vi "add_customize_control.vi"(8 "error in":errorcluster, 9 "Control Path":path, 10 "Control Position on BD":cluster{"Left":i32, "Top":i32}, 11 "VI Ref In":refnum<vi>) -> (0 "error out":errorcluster, 2 "Ctl Refnum":refnum<vi>, 3 "VI Ref Out":refnum<vi>)   [LabVIEW 2018]
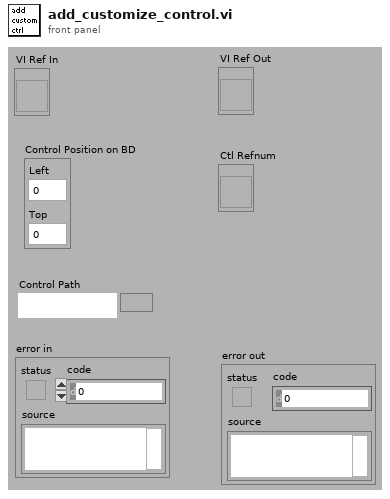
[diagram p1: front panel]
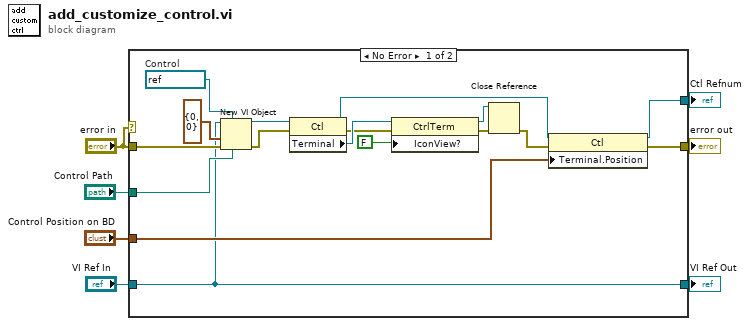
[diagram p0: block diagram]
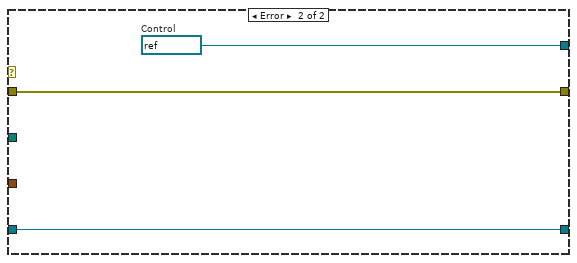
[diagram p2: hidden frame]
diagram:
  n1 = case shown="No Error" "error in" {
    tunnel: "Control Position on BD" -> [w24 _]
    tunnel: [w23 w27] -> w6
    tunnel: [w22 w26] -> w5
    tunnel: "VI Ref In" -> [w17 w25]
    tunnel: "Control Path" -> [w19 _]
    tunnel: "error in" -> [w18 w27]
    tunnel: [w17 w25] -> w1
    frame No Error {
      w21 = refnum<vi> refnum  # Control
      n2 = New VI Object(vi object class=w21, owner refnum=w17, position/next to=cluster{"Horizontal":i16, "Vertical":i16} {"Horizontal"=0, "Vertical"=0}, 6:w19, 8:w18) -> (object refnum=w11:refnum<vi>, 0:w10:errorcluster)  [unwired: 1 in, 2 out]
      n3 = property class="Ctl"(reference=w11, error in=w10) -> (reference out=w8:refnum<vi>, error out=w12:errorcluster, "Terminal"=w13:refnum<vi>)
      n4 = property class="CtrlTerm"(reference=w13, error in=w12, "IconView?"=FALSE ("Icon View?")) -> (reference out=w15:refnum<vi>, error out=w16:errorcluster)
      n5 = Close Reference(reference=w15, error in (no error)=w16) -> (error out=w9:errorcluster)
      n6 = property class="Ctl"(reference=w8, error in=w9, "Terminal.Position"=w24) -> (reference out=w22:refnum<vi>, error out=w23:errorcluster)
    }
    frame Error {
      w26 = refnum<vi> refnum  # Control
    }
  }
  "error out" <- w6
  "Ctl Refnum" <- w5
  "VI Ref Out" <- w1
